vi "Filter.vi"(8 "error in (no error)":errorcluster caption="错误输入（无错误）", 11 "O-Waveform输入":waveform(dbl)) -> (0 "error out":errorcluster caption="错误输出", 3 "F_Waveform输出":waveform(dbl))   [LabVIEW 2019]
uses:
  <vilib>/measure/matone.llb/Harmonic Distortion Analyzer 1 Chan.vi
  <vilib>/Analysis/3filter.llb/Butterworth Filter (DBL).vi
  <vilib>/measure/NI_MAPro.lvlib
  <vilib>/Analysis/NI_AALBase.lvlib
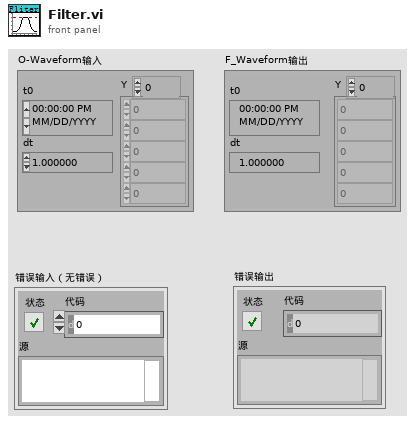
[diagram p1: front panel]
types:
  T1 = enum32{"Lowpass", "Highpass", "Bandpass", "Bandstop"}
  T2 = cluster{"approx freq. (optional)":dbl, "search (+/- % of Fsampl.)":dbl}
  T3 = enum16{"none", "input signal", "fundamental signal", "residual signal"}
  T4 = cluster{"exported time signal":waveform(dbl), "exported spectrum (dB)":cluster{"f0":dbl, "df":dbl, "dB Spectrum (Hann)":dbl[]}}
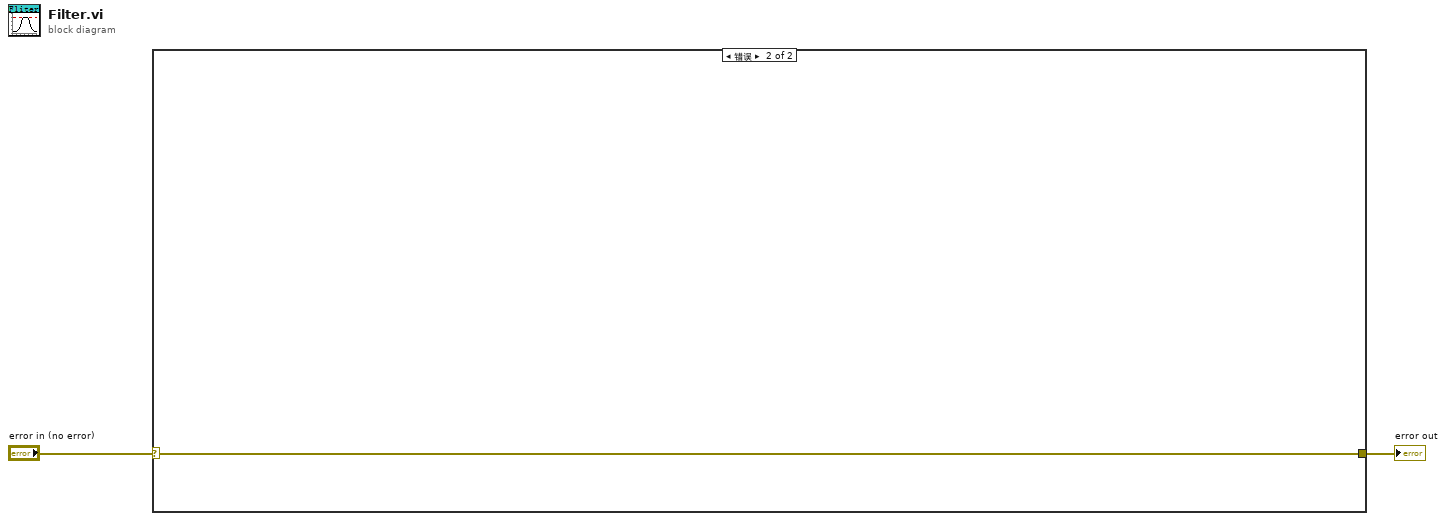
[diagram p0: block diagram]
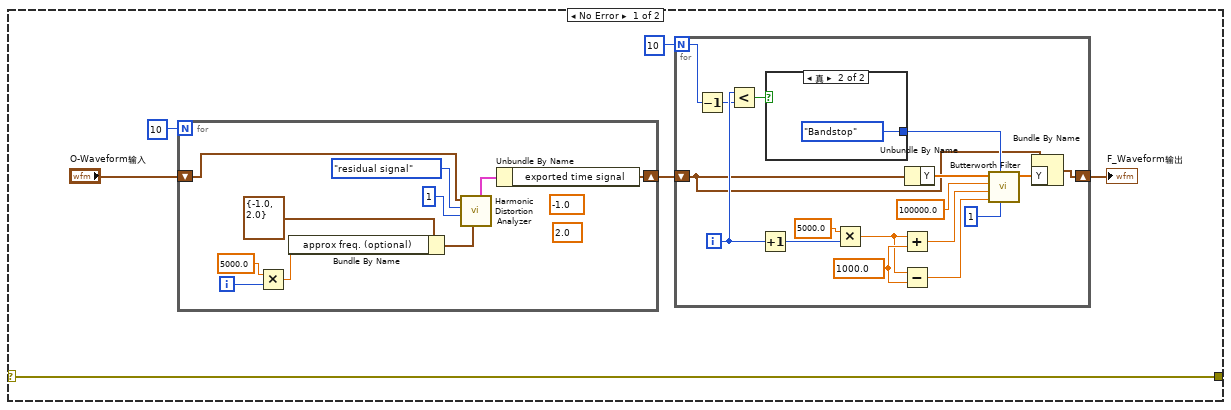
[diagram p2: hidden frame]
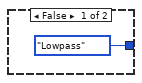
[diagram p3: hidden frame]
diagram:
  n1 = case shown="错误" "error in (no error)" {
    selector: "error in (no error)" -> [w3 w38]
    tunnel: [w3 w38] -> w1
    frame No Error {
      n2 = for {
        N: 10 -> [_]
        shift-right: [w31] -> w6
        shift-left: "O-Waveform输入" -> [w33]
        i -> [w30]
        (unwired) -1.0 ("approx freq. (optional)")
        (unwired) 2.0 ("search (+/- % of Fsampl.)")
        n3 = Multiply(x=5000.0, y=w30) -> (x*y=w32:dbl)
        n4 = Bundle By Name(cluster=T2 {"approx freq. (optional)"=-1.0, "search (+/- % of Fsampl.)"=2.0} ("advanced search"), "approx freq. (optional)"=w32) -> (w34:T2)
        n5 = call-poly <vilib>:"Harmonic Distortion Analyzer.vi"("advanced search"=w34, "highest harmonic"=1, "export mode"=T3."residual signal" ("export signals"), "signal in"=w33) -> ("exported signals"=w36:T4)  [unwired: 2 in, 5 out]
        n6 = Unbundle By Name(w36) -> ("exported time signal"=w31:waveform(dbl))
      }
      n7 = for {
        N: 10 -> [w11]
        shift-right: [w14] -> w8
        shift-left: w6 -> [w13]
        i -> [w16]
        w19 = 1000.0 ("high cutoff freq: fh")
        n8 = Decrement(x=w11) -> (x-1=w12:i32)
        n9 = Less?(x=w16, y=w12) -> (x < y?=w15:bool)
        n10 = Increment(x=w16) -> (x+1=w17:i32)
        n11 = case shown="真" w15 {
          tunnel: [T1."Lowpass" ("filter type") T1."Bandstop" ("filter type")] -> w25
          frame False {
          }
          frame True {
          }
        }
        n12 = Multiply(x=5000.0, y=w17) -> (x*y=w18:dbl)
        n13 = Add(x=w18, y=w19) -> (x+y=w20:dbl)
        n14 = Subtract(x=w18, y=w19) -> (x-y=w21:dbl)
        n15 = Unbundle By Name(w13) -> ("Y"=w22:dbl[])
        n16 = call-poly <vilib>:"Butterworth Filter.vi"("order"=1, "filter type"=w25, "low cutoff freq: fl"=w21, "high cutoff freq: fh"=w20, "sampling freq: fs"=100000.0, "X"=w22) -> ("Filtered X"=w23:dbl[])  [unwired: 2 in, 1 out]
        n17 = Bundle By Name(cluster=w13, "Y"=w23) -> (w14:waveform(dbl))
      }
      "F_Waveform输出" <- w8
    }
    frame Error {
    }
  }
  "error out" <- w1
